vi "DiffDriveKinematicsConstraint_getMaxVelocity.vi"(8 "Velocity":dbl, 9 "Curvature":dbl, 10 "statePose":T3={"TRANSLATION"={"X"=0.0, "Y"=0.0}, "ROTATION"={"VALUE"=0.0, "COS"=1.0, "SIN"=0.0}} {"ROTATION"."SIN" format="%13.4f"; "ROTATION"."COS" format="%13.4f"; "ROTATION"."VALUE" format="%13.4f"; "TRANSLATION"."Y" format="%14.3f"; "TRANSLATION"."X" format="%14.3f"}, 11 "DIFF_DRIVE_KINE_CONSTRAINT":T1={"Max Speed (M/S)"=0.0, "DIFF_DRIVE_KINEMATICS"={"TrackWidth_Meters"=0.0}, "Max Accel (M/S2)"=99999.0} {"Max Accel (M/S2)" format="%20.4f"; "DIFF_DRIVE_KINEMATICS"."TrackWidth_Meters" format="%20.4f"; "Max Speed (M/S)" format="%20.4f"}) -> (3 "absMaxVelocity":dbl)   [LabVIEW 2019, in "Trajectory_Library.lvlib"]
doc: "Return the maximum allowed velocity given the provided conditions.\n\nEnsure each individual normalized wheel speed is within the defined maximum velocity.\n\nParameters:\n - DiffDriveKinematicsConstraint - Constraint data structure\n - statePose - current traj state Pose\n - curvature - current traj curvature\n - maxVelocity - current traj max velocity\n\nReturns\n - maxVelocity - Maximum allowed velocity."
uses:
  Trajectory_Library.lvlib
  TypeDef/TRANSLATION2D.ctl
  TypeDef/ROTATION2D.ctl
  TypeDef/POSE2D.ctl
  TypeDef/DIFF_DRIVE_KINEMATICS.ctl
  TypeDef/TRAJ_CONSTRAINT_DIIF_DRIVE_KINEMATICS.ctl
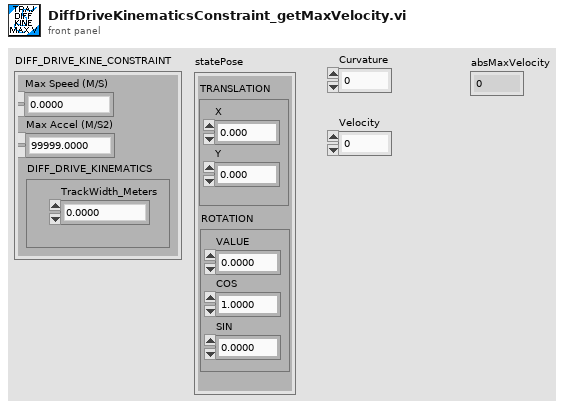
[diagram p1: front panel]
types:
  T1 = typedef "Trajectory_Library.lvlib/TRAJ_CONSTRAINT_DIIF_DRIVE_KINEMATICS.ctl" = cluster{"Max Speed (M/S)":dbl, "DIFF_DRIVE_KINEMATICS":T2, "Max Accel (M/S2)":dbl}
  T2 = typedef "Trajectory_Library.lvlib/DIFF_DRIVE_KINEMATICS.ctl" = cluster{"TrackWidth_Meters":dbl}
  T3 = typedef "Trajectory_Library.lvlib/POSE2D.ctl" = cluster{"TRANSLATION":T4, "ROTATION":T5}
  T4 = typedef "Trajectory_Library.lvlib/TRANSLATION2D.ctl" = cluster{"X":dbl, "Y":dbl}
  T5 = typedef "Trajectory_Library.lvlib/ROTATION2D.ctl" = cluster{"VALUE":dbl, "COS":dbl, "SIN":dbl}
  T6 = typedef "Trajectory_Library.lvlib/CHASSIS_SPEEDS.ctl" = cluster{"vX":dbl, "vY":dbl, "vOmega":dbl}
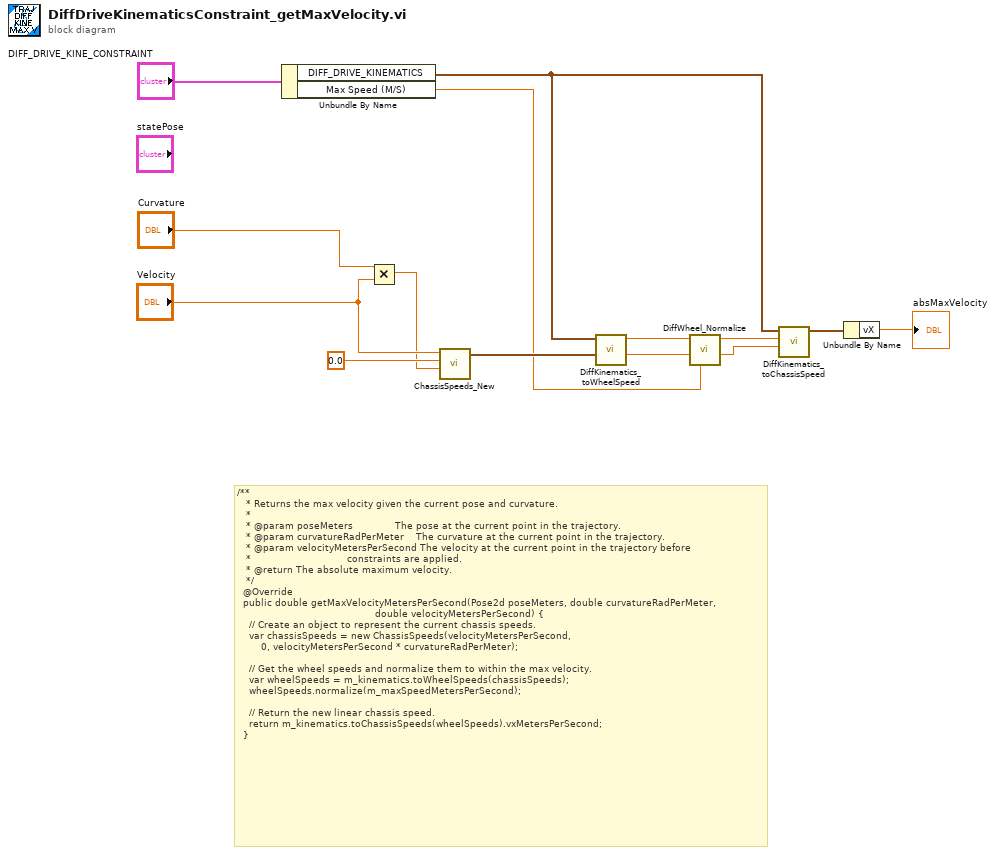
[diagram p0: block diagram]
diagram:
  # "/**\n   * Returns the max velocity given the current pose and curvature.\n   *\n   * @param poseMeters              The pose at the current point in the trajectory.\n   * @param curvatureRadPerMeter    The curvature at the current point in the trajectory.\n   * @param velocityMetersPerSecond The velocity at the current point in the trajectory before\n   *                                constraints are applied.\n   * @return The absolute maximum velocity.\n   */\n  @Override\n  public double getMaxVelocityMetersPerSecond(Pose2d poseMeters, double curvatureRadPerMeter,\n                                              double velocityMetersPerSecond) {\n    // Create an object to represent the current chassis speeds.\n    var chassisSpeeds = new ChassisSpeeds(velocityMetersPerSecond,\n        0, velocityMetersPerSecond * curvatureRadPerMeter);\n\n    // Get the wheel speeds and normalize them to within the max velocity.\n    var wheelSpeeds = m_kinematics.toWheelSpeeds(chassisSpeeds);\n    wheelSpeeds.normalize(m_maxSpeedMetersPerSecond);\n\n    // Return the new linear chassis speed.\n    return m_kinematics.toChassisSpeeds(wheelSpeeds).vxMetersPerSecond;\n  }"
  n1 = Unbundle By Name("DIFF_DRIVE_KINE_CONSTRAINT") -> ("DIFF_DRIVE_KINEMATICS"=w6:T2, "Max Speed (M/S)"=w7:dbl)
  n2 = Multiply(x="Curvature", y="Velocity") -> (x*y=w11:dbl)
  n3 = call "ChassisSpeeds_New.vi"("vAngular"=w11, "vY"=0.0, "vX"="Velocity") -> ("CHASSIS"=w10:T6)  [unwired: 8 in]
  n4 = call "DiffKinematics_toWheelSpeed.vi"("CHASSIS Speed"=w10, "DIFF_DRIVE_KINEMATICS"=w6) -> ("RightVelocity"=w8:dbl, "LeftVelocity"=w9:dbl)  [unwired: 8 in]
  n5 = call "DiffWheel_Normalize.vi"("Max Speed"=w7, "Right Wheel Demand"=w8, "Left Wheel Demand"=w9) -> ("Normalized Right Wheel Demand"=w4:dbl, "Normalized Left Wheel Demand"=w5:dbl)  [unwired: 7 in]
  n6 = call "DiffKinematics_toChassisSpeed.vi"("RightVelocity"=w4, "LeftVelocity"=w5, "inDIFF_DRIVE_KINEMATICS"=w6) -> ("CHASSIS Speed"=w3:T6)  [unwired: 8 in]
  n7 = Unbundle By Name(w3) -> ("vX"=→"absMaxVelocity":dbl)
